vi "Lang Set Other.vi"(8 "error in (no error)":errorcluster, 10 "Other":T1, 11 "LF2R IDE in":refnum<class "Main Panel.lvclass">) -> (0 "error out":errorcluster, 3 "LF2R IDE out":refnum<class "Main Panel.lvclass">)   [LabVIEW 2018, in "Main Panel.lvlib" / "Main Panel.lvclass"]
uses:
  Main Panel.lvclass
  Framework/Framework/Const Lang MainWnd Other.ctl
  Framework/Framework/Const Lang Property.ctl
  Main Panel.lvclass/Main Panel.ctl
  Framework/Framework/Framework.lvclass
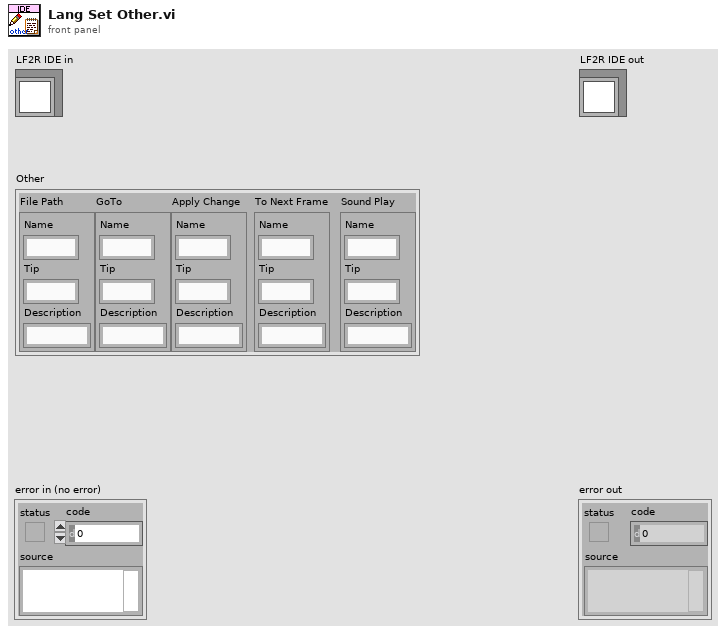
[diagram p1: front panel]
types:
  T1 = typedef "Framework.lvlib/Framework.lvclass/Const Lang MainWnd Other.ctl" = cluster{"File Path":T2, "GoTo":T2, "Apply Change":T2, "To Next Frame":T2, "Sound Play":T2}
  T2 = typedef "Framework.lvlib/Framework.lvclass/Const Lang Property.ctl" = cluster{"Name":string, "Tip":string, "Description":string}
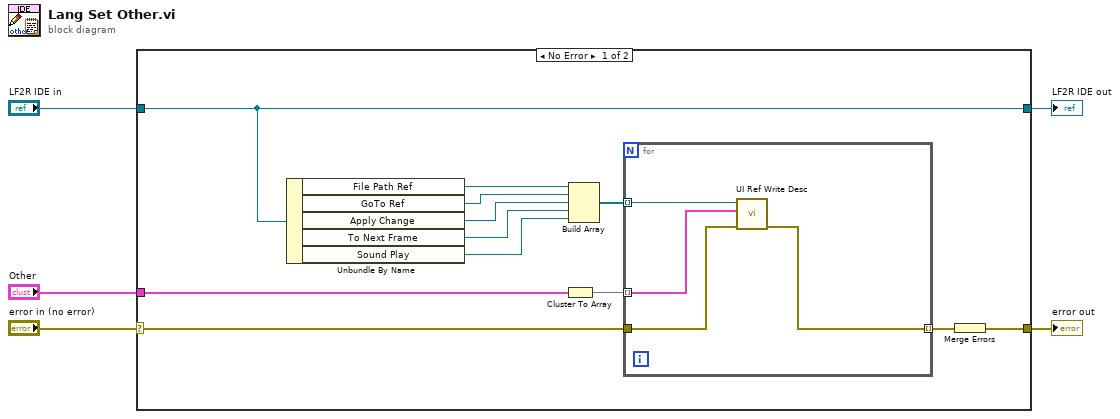
[diagram p0: block diagram]
diagram:
  n1 = case shown="No Error" "error in (no error)" {
    selector: "error in (no error)" -> [w15 w23]
    tunnel: [w14 w23] -> w4
    tunnel: [w17 w22] -> w2
    tunnel: "LF2R IDE in" -> [w17 w22]
    tunnel: "Other" -> [w16 _]
    frame No Error {
      n2 = Unbundle By Name(w17) -> ("File Path Ref"=w10:refnum<vi>, "GoTo Ref"=w9:refnum<vi>, "Apply Change"=w8:refnum<vi>, "To Next Frame"=w7:refnum<vi>, "Sound Play"=w6:refnum<vi>)
      n3 = Cluster To Array(cluster=w16) -> (array=w12:T2[])
      n4 = Build Array(w10, w9, w8, w7, w6) -> (w13:refnum<vi>[])
      n5 = for {
        tunnel: w13 -> [w18] mode=indexing
        tunnel: w12 -> [w21] mode=indexing
        tunnel: w15 -> [w20]
        tunnel: [w19] -> w11 mode=indexing
        n6 = call "UI Ref Write Desc.vi"("error in (no error)"=w20, "UI Property"=w21, "UI Ref"=w18) -> ("error out"=w19:errorcluster)  [unwired: 8 in]
      }
      n7 = Merge Errors(w11) -> (w14:errorcluster)
    }
    frame Error {
    }
  }
  "error out" <- w4
  "LF2R IDE out" <- w2
